vi "Editor UI.vi"(8 "error in (no error)":errorcluster, 11 "Entity Editor in":refnum<class "Entity Editor.lvclass">) -> (0 "error out":errorcluster, 3 "Entity Editor out":refnum<class "Entity Editor.lvclass">)   [LabVIEW 2020, in "Conditum-Tools.lvlib" / "Entity Editor.lvclass"]
uses:
  Entity Editor.lvclass
  Conditum-Clone/Columns/Type/Type.lvclass
  ColumnPanel/ColumnPanel.lvclass
  C:/Program Files (x86)/National Instruments/LabVIEW 2020/vi.lib/IlluminatedG/IG OOPanel/OOPanel/ArrayPanel/ArrayPanel.lvclass
  Conditum-Clone/Columns/Type/Type.lvclass/Type.ctl
  <vilib>/IlluminatedG/IG OOPanel/OOPanel/ArrayManager/ArrayManager.lvclass
  1c4234d0-757c-494a-9175-61bb4fd4687c.vi
  2443108f-0f49-4029-b3c0-d61e9c764f54.vi
  <vilib>/Utility/cursorutil.llb/Set Cursor (Icon Pict).vi
  <vilib>/Utility/LVClass/Get LV Class Name.vi
  <vilib>/Comparison/Equal/Equal Functor/Equal Functor.lvclass
panel:
  out "Project Ref":refnum<vi>
  out "Entity Path":path
  in  "Reset Entity":bool
  in  "Save Entity":bool
  in  "Fields":i32(listbox)
  out "Definition":refnum<class "Type.lvclass">[](array[class])
  out "Target Entity Paths":path[](array[path])
  in  "Refresh Targets":bool
  in  "Target":string(combo)
  in  "Refresh Projects":bool
  in  "New Entity":bool
  in  "Remove Field":bool
  in  "Add Field":bool
  in  "Entity":i32(listbox)
  in  "Project":string(combo)
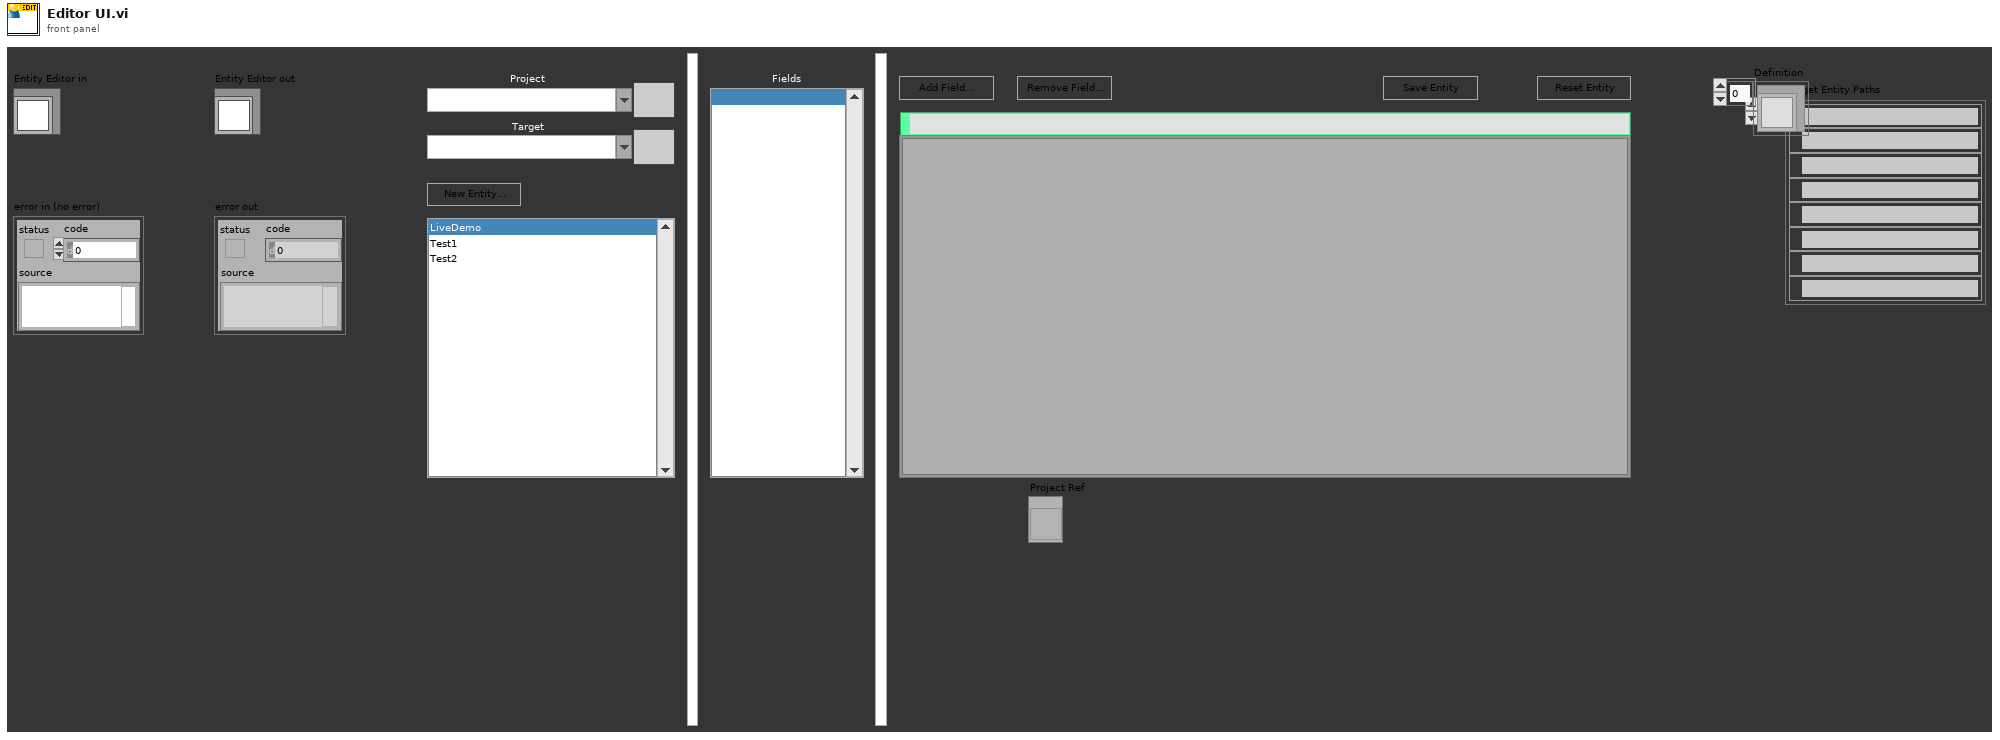
[diagram p1: front panel]
types:
  T1 = typedef "Conditu2.lvlib/Field Type.ctl" = enum16{"None", "ID", "Boolean", "Integer", "Double", "Timestamp", "String", "Text", "Entity"}
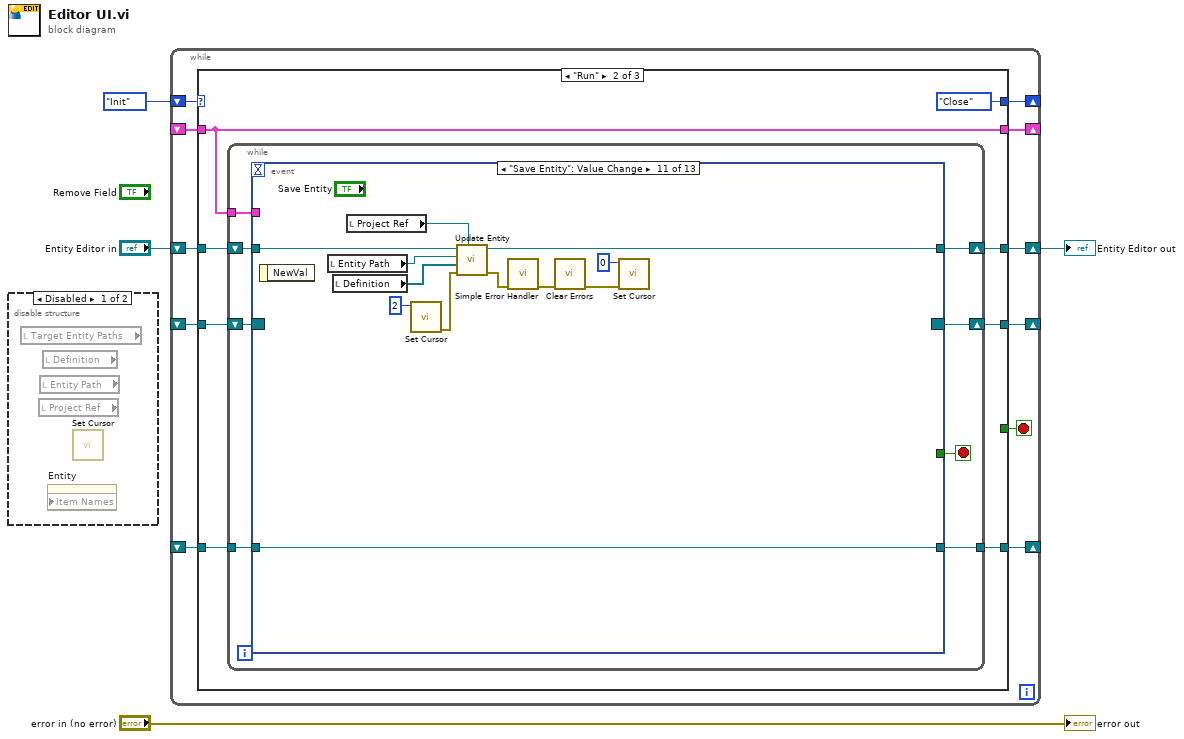
[diagram p0: block diagram]
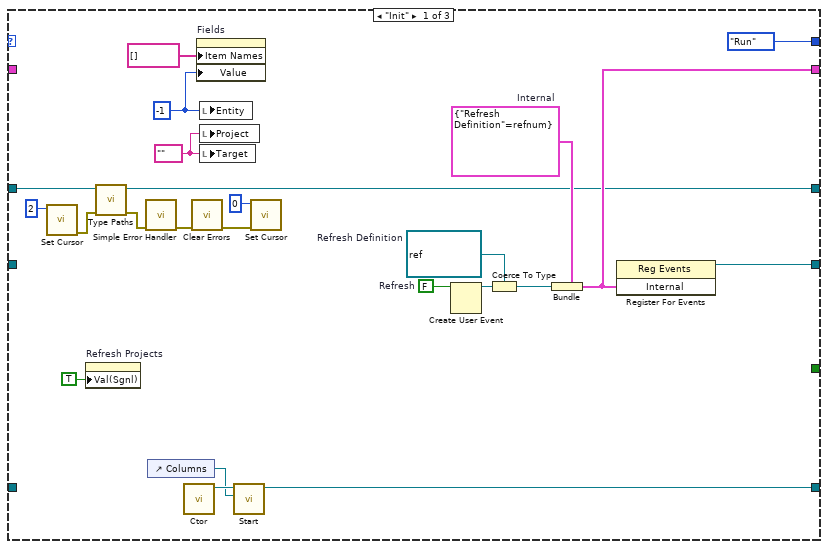
[diagram p3: hidden frame]
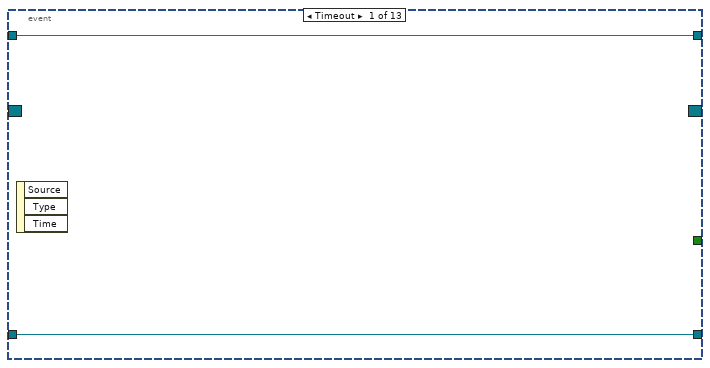
[diagram p4: hidden frame]
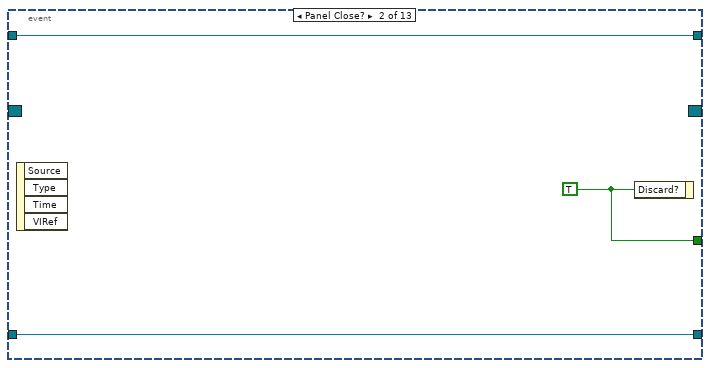
[diagram p5: hidden frame]
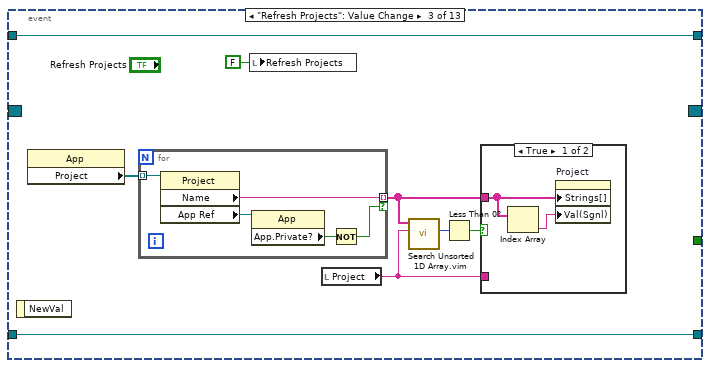
[diagram p6: hidden frame]
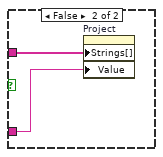
[diagram p7: hidden frame]
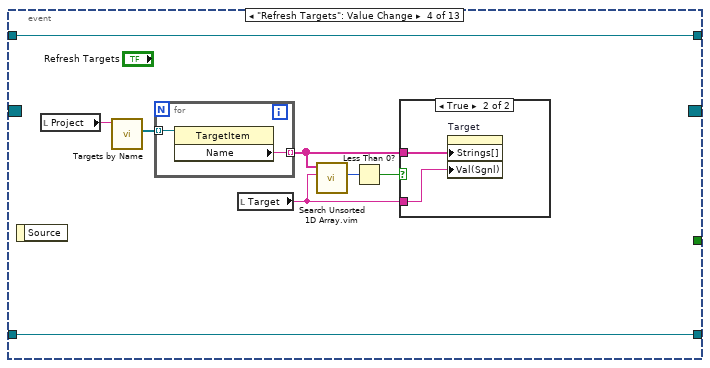
[diagram p8: hidden frame]
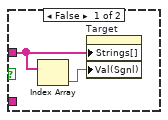
[diagram p9: hidden frame]
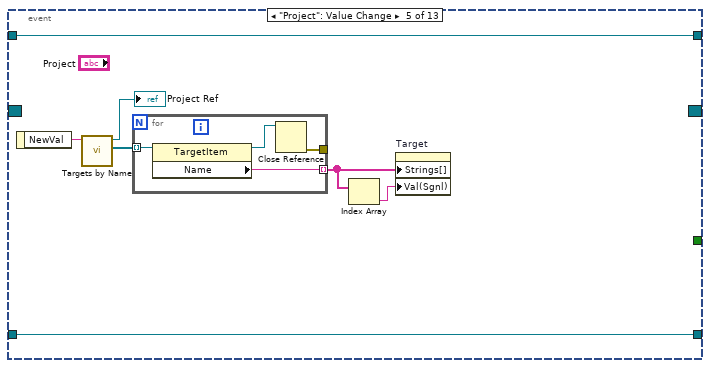
[diagram p10: hidden frame]
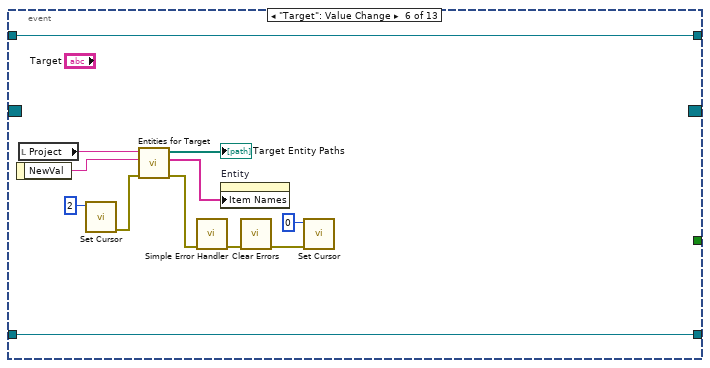
[diagram p11: hidden frame]
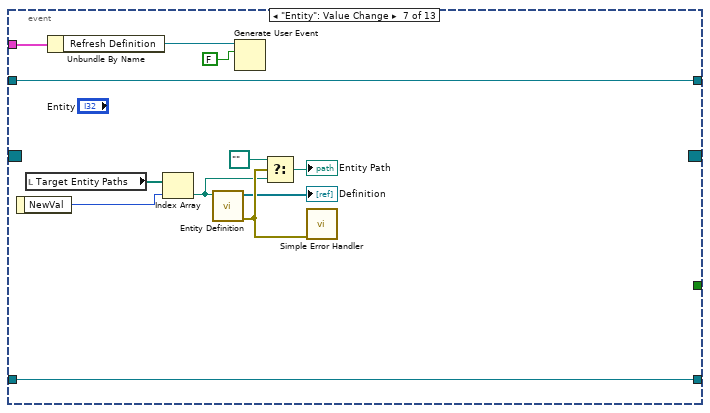
[diagram p12: hidden frame]
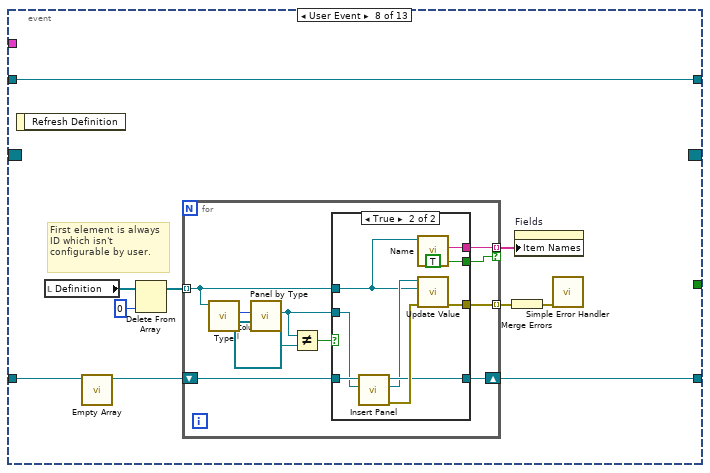
[diagram p13: hidden frame]
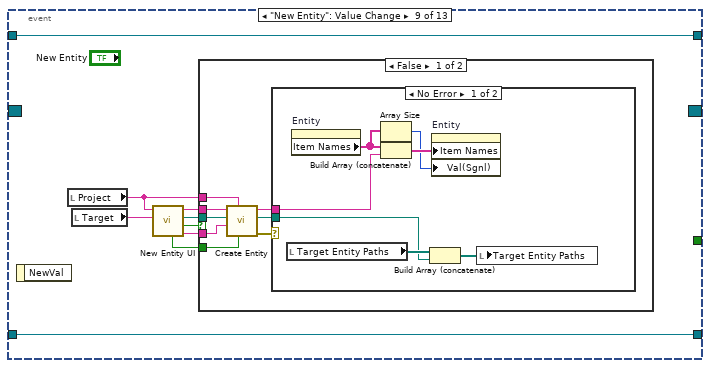
[diagram p15: hidden frame]
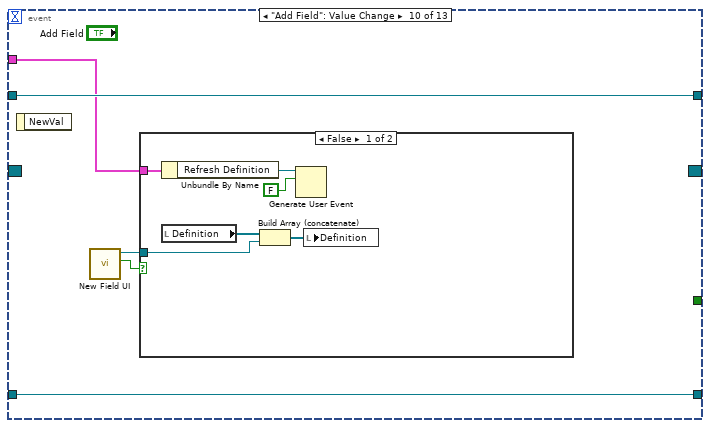
[diagram p18: hidden frame]
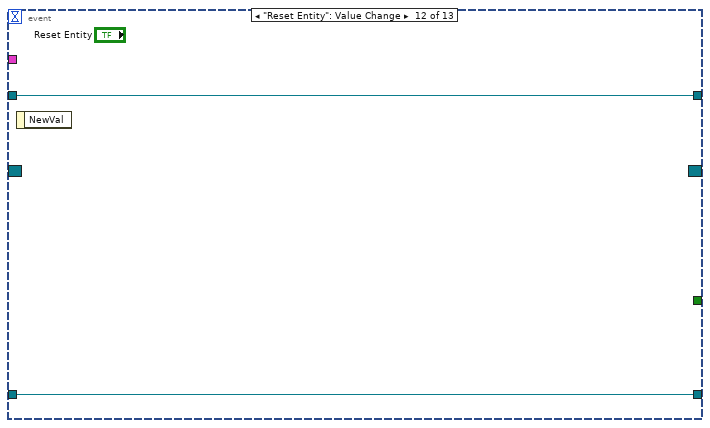
[diagram p20: hidden frame]
diagram:
  n1 = disable-structure shown="Disabled" {
    frame Disabled {
      n2 = local read "Target Entity Paths"() -> ()  [unwired: 1 out]
      n3 = local read "Project Ref"() -> ()  [unwired: 1 out]
      n4 = local read "Entity Path"() -> ()  [unwired: 1 out]
      n5 = local read "Definition"() -> ()  [unwired: 1 out]
      n6 = property on="Entity" class="LstBox (strict)" props=["Item Names"]() -> ()  [unwired: 3 in, 2 out]
      n7 = call-poly <vilib>:"Set Cursor.vi"() -> ()  [unwired: 10 in, 2 out]
    }
    frame Enabled {
    }
  }
  n8 = while {
    shift-right: [w14] -> _
    shift-left: enum16{"Init", "Run", "Close"}."Init" ("Basic UI State") -> [w15]
    shift-right: [w12] -> w2
    shift-left: "Entity Editor in" -> [w13]
    shift-right: [w10] -> _
    shift-left: _ -> [w9]
    shift-right: [w8] -> _
    shift-left: _ -> [w7]
    shift-right: [w6] -> _
    shift-left: _ -> [w5]
    stop <- w11 stop-if-true
    n9 = case shown="\"Run\"" w15 {
      selector: w15 -> [_ _ w216]
      tunnel: [enum16{"Init", "Run", "Close"}."Run" ("Basic UI State") enum16{"Init", "Run", "Close"}."Close" ("Basic UI State") w216] -> w14
      tunnel: w13 -> [w24 w45 w215]
      tunnel: [w23 w44 w215] -> w12
      tunnel: [_ _ TRUE] -> w11
      tunnel: [w31 w42 refnum<class "ArrayManager.lvclass"> refnum ("ArrayManager out")] -> w10
      tunnel: w9 -> [_ w43 w213]
      tunnel: [w27 w40 _] -> w8
      tunnel: w7 -> [_ w41 w209]
      tunnel: [w28 w39 _] -> w6
      tunnel: w5 -> [_ w39 w211]
      frame "Init" {
        w21 = "" ("Target")
        w25 = -1 ("Entities")
        w29 = cluster{"Refresh Definition":refnum<user-event>} {"Refresh Definition"=refnum}  # Internal
        w33 = refnum<user-event> refnum  # Refresh Definition
        w35 = FALSE  # Refresh
        n10 = call-poly <vilib>:"Set Cursor.vi"("icon"=u16 2) -> ("error out"=w19:errorcluster)  [unwired: 9 in, 1 out]
        n11 = property on="Refresh Projects" class="Bool (strict)"("Val(Sgnl)"=TRUE ("Value (Signaling)")) -> ()  [unwired: 2 in, 2 out]
        n12 = call "Type Paths.vi"("error in (no error)"=w19, "Editor in"=w24) -> ("error out"=w22:errorcluster, "Editor out"=w23:refnum<class "Entity Editor.lvclass">)  [unwired: 8 in]
        n13 = call <vilib>:"Simple Error Handler.vi"("error in (no error)"=w22) -> ("error out"=w18:errorcluster)  [unwired: 4 in, 4 out]
        n14 = control-ref of="Columns"() -> (w36:refnum<vi>)
        n15 = call <vilib>:"Ctor.vi"() -> ("PanelArray"=w37:refnum<class "ArrayManager.lvclass">)  [unwired: 10 in, 1 out]
        n16 = call <vilib>:"Clear Errors.vi"("error in (no error)"=w18) -> ("error out"=w17:errorcluster)  [unwired: 5 in, 1 out]
        n17 = property on="Fields" class="LstBox (strict)"("Item Names"=string[] [], "Value"=w25) -> ()  [unwired: 2 in, 2 out]
        n18 = local write "Entity"(w25) -> ()
        n19 = local write "Project"(w21) -> ()
        n20 = local write "Target"(w21) -> ()
        n21 = call <vilib>:"Start.vi"("Container"=w36, "ArrayManager in"=w37) -> ("ArrayManager out"=w31:refnum<class "ArrayManager.lvclass">)  [unwired: 8 in, 1 out]
        n22 = call-poly <vilib>:"Set Cursor.vi"("error in (no error)"=w17, "icon"=u16 0) -> ()  [unwired: 8 in, 2 out]
        n23 = Create User Event(user event datatype=w35) -> (user event=w34:refnum<user-event>)  [unwired: 1 in, 1 out]
        n24 = Coerce To Type(0:w34, 1:w33) -> (2:w32:refnum<user-event>)
        n25 = Bundle(cluster=w29, "Refresh Definition"=w32) -> (w28:cluster{"Refresh Definition":refnum<user-event>})
        n26 = register-events(w28) -> (reference out=w27:refnum<event-registration>)  [unwired: 2 in, 1 out]
      }
      frame "Run" {
        n27 = while {
          shift-right: [w54] -> w44
          shift-left: w45 -> [w53]
          tunnel: w43 -> [w51]
          tunnel: [w50] -> w42
          shift-right: [w49] -> w40
          shift-left: w41 -> [w47]
          tunnel: w39 -> [w48]
          stop <- w52 stop-if-true
          n28 = event shown="[10] \"Save Entity\": Value Change" {
            selector: w47 -> [_ _ _ _ _ _ _ _ _ _ _ _ _]
            dyn-events: [_ _ _ _ _ _ _ _ _ _ _ _ _] -> w49
            timeout: _ -> [_ _ _ _ _ _ _ _ _ _ _ _ _]
            tunnel: [w56 w59 w67 w84 w97 w113 w124 w135 w161 w181 w200 w204 w208] -> w54
            tunnel: w53 -> [w56 w59 w67 w84 w97 w113 w124 w135 w161 w181 w201 w204 w208]
            tunnel: [_ w58 _ _ _ _ _ _ _ _ _ _ _] -> w52
            tunnel: w51 -> [w55 w57 w66 w83 w96 w112 w123 w131 w164 w184 w202 w203 w206]
            tunnel: [w55 w57 w66 w83 w96 w112 w123 w129 w164 w184 w202 w203 w206] -> w50
            tunnel: w48 -> [_ _ _ _ _ _ w120 _ _ w180 _ _ _]
            event Timeout {
              n29 = event-data() -> ()  [unwired: 1 in, 3 out]
            }
            event Panel Close? {
              w58 = TRUE ("Discard?")
              n30 = event-data() -> ()  [unwired: 1 in, 4 out]
              n31 = event-data("Discard?"=w58) -> ()  [unwired: 1 in, 1 out]
            }
            event "Refresh Projects": Value Change {
              n32 = event-data() -> ()  [unwired: 1 in, 1 out]
              n33 = property class="App"() -> ("Project"=w64:refnum<vi>[])  [unwired: 2 in, 2 out]
              n34 = for {
                tunnel: w64 -> [w76] mode=indexing
                tunnel: [w73] -> w63 mode=indexing if=w72
                n35 = property class="Project"(reference=w76) -> ("Name"=w73:string, "App Ref"=w75:refnum<vi>)  [unwired: 1 in, 2 out]
                n36 = property class="App"(reference=w75) -> ("App.Private?"=w74:bool)  [unwired: 1 in, 2 out]
                n37 = Not(x=w74) -> (.not. x?=w72:bool)
              }
              n38 = local write "Refresh Projects"(FALSE ("Refresh Projects")) -> ()
              n39 = local read "Project"() -> (w60:string)
              n40 = call "Search Unsorted 1D Array.vim"("element"=w60, "unsorted 1D array"=w63) -> ("index of element"=w62:i32)  [unwired: 9 in]
              n41 = Less Than 0?(x=w62) -> (x < 0?=w61:bool)
              n42 = case shown="True" w61 {
                tunnel: w63 -> [w69 w71]
                tunnel: w60 -> [_ w70]
                frame True {
                  n43 = Index Array(array=w69) -> (element=w68:string)  [unwired: 1 in]
                  n44 = property on="Project" class="CmbBox"("Strings[]"=w69, "Val(Sgnl)"=w68) -> ()  [unwired: 2 in, 2 out]
                }
                frame False {
                  n45 = property on="Project" class="CmbBox"("Strings[]"=w71, "Value"=w70) -> ()  [unwired: 2 in, 2 out]
                }
              }
            }
            event "Refresh Targets": Value Change {
              n46 = event-data() -> ()  [unwired: 1 in, 1 out]
              n47 = local read "Project"() -> (w81:string)
              n48 = call "Targets by Name.vi"("Project Name"=w81) -> ("Targets"=w82:refnum<vi>[])  [unwired: 9 in, 1 out]
              n49 = for {
                tunnel: w82 -> [w90] mode=indexing
                tunnel: [w89] -> w78 mode=indexing
                n50 = property class="TargetItem"(reference=w90) -> ("Name"=w89:string)  [unwired: 1 in, 2 out]
              }
              n51 = local read "Target"() -> (w77:string)
              n52 = call "Search Unsorted 1D Array.vim"("element"=w77, "unsorted 1D array"=w78) -> ("index of element"=w80:i32)  [unwired: 9 in]
              n53 = Less Than 0?(x=w80) -> (x < 0?=w79:bool)
              n54 = case shown="True" w79 {
                tunnel: w78 -> [w86 w88]
                tunnel: w77 -> [_ w87]
                frame False {
                  n55 = Index Array(array=w86) -> (element=w85:string)  [unwired: 1 in]
                  n56 = property on="Target" class="CmbBox"("Strings[]"=w86, "Val(Sgnl)"=w85) -> ()  [unwired: 2 in, 2 out]
                }
                frame True {
                  n57 = property on="Target" class="CmbBox"("Strings[]"=w88, "Val(Sgnl)"=w87) -> ()  [unwired: 2 in, 2 out]
                }
              }
            }
            event "Project": Value Change {
              n58 = event-data() -> ("NewVal"=w95:string)  [unwired: 1 in]
              n59 = call "Targets by Name.vi"("Project Name"=w95) -> ("Targets"=w94:refnum<vi>[], "Project"=→"Project Ref":refnum<vi>)  [unwired: 9 in]
              n60 = for {
                tunnel: w94 -> [w101] mode=indexing
                tunnel: [w100] -> w93 mode=indexing
                tunnel: [w98] -> _
                n61 = property class="TargetItem"(reference=w101) -> (reference out=w99:refnum<vi>, "Name"=w100:string)  [unwired: 1 in, 1 out]
                n62 = Close Reference(reference=w99) -> (error out=w98:errorcluster)  [unwired: 1 in]
              }
              n63 = Index Array(array=w93) -> (element=w92:string)  [unwired: 1 in]
              n64 = property on="Target" class="CmbBox"("Strings[]"=w93, "Val(Sgnl)"=w92) -> ()  [unwired: 2 in, 2 out]
            }
            event "Target": Value Change {
              n65 = event-data() -> ("NewVal"=w110:string)  [unwired: 1 in]
              n66 = local read "Project"() -> (w111:string)
              n67 = call-poly <vilib>:"Set Cursor.vi"("icon"=u16 2) -> ("error out"=w106:errorcluster)  [unwired: 9 in, 1 out]
              n68 = call "Entities for Target.vi"("error in (no error)"=w106, "Target Name"=w110, "Project Name"=w111) -> ("error out"=w107:errorcluster, "Names"=w108:string[], "Entities"=→"Target Entity Paths":path[])  [unwired: 6 in]
              n69 = call <vilib>:"Simple Error Handler.vi"("error in (no error)"=w107) -> ("error out"=w104:errorcluster)  [unwired: 4 in, 4 out]
              n70 = property on="Entity" class="LstBox (strict)"("Item Names"=w108) -> ()  [unwired: 2 in, 2 out]
              n71 = call <vilib>:"Clear Errors.vi"("error in (no error)"=w104) -> ("error out"=w102:errorcluster)  [unwired: 5 in, 1 out]
              n72 = call-poly <vilib>:"Set Cursor.vi"("error in (no error)"=w102, "icon"=u16 0) -> ()  [unwired: 8 in, 2 out]
            }
            event "Entity": Value Change {
              n73 = event-data() -> ("NewVal"=w121:i32)  [unwired: 1 in]
              n74 = local read "Target Entity Paths"() -> (w122:path[])
              n75 = Unbundle By Name(w120) -> ("Refresh Definition"=w119:refnum<user-event>)
              n76 = Index Array(array=w122, index=w121) -> (element=w116:path)
              n77 = call "Entity Definition.vi"("Path"=w116) -> ("error out"=w125:errorcluster, "Definition"=→"Definition":refnum<class "Type.lvclass">[])  [unwired: 8 in, 1 out]
              n78 = Generate User Event(user event=w119, event data cluster=FALSE ("event data")) -> ()  [unwired: 2 in, 2 out]
              n79 = Select(t=path "", s=w125, f=w116) -> (s? t:f=→"Entity Path":path)
              n80 = call <vilib>:"Simple Error Handler.vi"("error in (no error)"=w125) -> ()  [unwired: 4 in, 5 out]
            }
            event User Event {
              # "First element is always ID which isn't configurable by user."
              n81 = event-data() -> ()  [unwired: 1 in, 1 out]
              n82 = local read "Definition"() -> (w134:refnum<class "Type.lvclass">[])
              n83 = call <vilib>:"Empty Array.vi"("ArrayManager in"=w131) -> ("ArrayManager out"=w130:refnum<class "ArrayManager.lvclass">)  [unwired: 9 in, 1 out]
              n84 = Delete From Array(array=w134, index=0) -> (array with subset deleted=w133:refnum<class "Type.lvclass">[])  [unwired: 1 in, 1 out]
              n85 = for {
                tunnel: w133 -> [w140] mode=indexing
                shift-right: [w139] -> w129
                shift-left: w130 -> [w143]
                tunnel: [w138] -> w128 mode=indexing
                tunnel: [w137] -> w126 mode=indexing if=w136
                n86 = call "Type.vi"("Type in"=w140) -> ("Type"=w145:T1)  [unwired: 10 in]
                n87 = call "Panel by Type.vi"("Type"=w145) -> ("ColumnPanel"=w141:refnum<class "ColumnPanel.lvclass">)  [unwired: 10 in]
                n88 = Not Equal?(x=w141, y=refnum<class "ColumnPanel.lvclass"> refnum) -> (x != y?=w142:bool)
                n89 = case shown="True" w142 {
                  tunnel: w143 -> [w146 w154]
                  tunnel: w141 -> [_ w153]
                  tunnel: w140 -> [_ w149]
                  tunnel: [w146 w152] -> w139
                  tunnel: [_ w151] -> w138
                  tunnel: [_ w148] -> w137
                  tunnel: [_ TRUE] -> w136
                  frame False {
                  }
                  frame True {
                    n90 = call <vilib>:"Insert Panel.vi"("Panel/Type"=w153, "PanelArray in"=w154) -> ("error out"=w155:errorcluster, "Panel"=w150:refnum<class "ColumnPanel.lvclass">, "PanelArray out"=w152:refnum<class "ArrayManager.lvclass">)  [unwired: 7 in]
                    n91 = call "Name.vi"("Type in"=w149) -> ("Table Name"=w148:string)  [unwired: 10 in]
                    n92 = call "Update Value.vi"("error in (no error)"=w155, "Type Value"=w149, "ColumnPanel in"=w150) -> ("error out"=w151:errorcluster)  [unwired: 7 in, 1 out]
                  }
                }
              }
              n93 = Merge Errors(w128) -> (w127:errorcluster)
              n94 = property on="Fields" class="LstBox (strict)"("Item Names"=w126) -> ()  [unwired: 2 in, 2 out]
              n95 = call <vilib>:"Simple Error Handler.vi"("error in (no error)"=w127) -> ()  [unwired: 4 in, 5 out]
            }
            event "New Entity": Value Change {
              n96 = event-data() -> ()  [unwired: 1 in, 1 out]
              n97 = local read "Project"() -> (w156:string)
              n98 = local read "Target"() -> (w162:string)
              n99 = call "New Entity UI.vi"("Target Name"=w162, "Project Name"=w156) -> ("Container"=w158:string, "Cancelled"=w160:bool, "Folder"=w159:path, "Entity Name"=w163:string, "Library?"=w157:bool)  [unwired: 5 in]
              n100 = case shown="False" w160 {
                tunnel: w163 -> [w167 _]
                tunnel: w159 -> [w172 _]
                tunnel: w158 -> [w171 _]
                tunnel: w157 -> [w169 _]
                tunnel: w156 -> [w170 _]
                frame False {
                  n101 = call "Create Entity.vi"("Library"=w169, "Project"=w170, "Container"=w171, "Folder"=w172, "Entity Name in"=w167) -> ("error out"=w168:errorcluster, "New Entity Path"=w165:path, "Entity Name"=w166:string)  [unwired: 4 in]
                  n102 = case shown="No Error" w168 {
                    tunnel: w166 -> [w179 _]
                    tunnel: w165 -> [w176 _]
                    frame No Error {
                      n103 = local read "Target Entity Paths"() -> (w177:path[])
                      n104 = property on="Entity" class="LstBox (strict)"() -> ("Item Names"=w174:string[])  [unwired: 2 in, 2 out]
                      n105 = Array Size(array=w174) -> (size(s)=w173:i32)
                      n106 = Build Array (concatenate)(w174, w179) -> (w178:string[])
                      n107 = Build Array (concatenate)(w177, w176) -> (w175:path[])
                      n108 = property on="Entity" class="LstBox (strict)"("Item Names"=w178, "Val(Sgnl)"=w173) -> ()  [unwired: 2 in, 2 out]
                      n109 = local write "Target Entity Paths"(w175) -> ()
                    }
                    frame Error {
                    }
                  }
                }
                frame True {
                }
              }
            }
            event "Add Field": Value Change {
              n110 = event-data() -> ()  [unwired: 1 in, 1 out]
              n111 = call "New Field UI.vi"() -> ("Cancelled"=w183:bool, "Field"=w182:refnum<class "Type.lvclass">)  [unwired: 10 in]
              n112 = case shown="False" w183 {
                tunnel: w182 -> [w189 _]
                tunnel: w180 -> [w187 _]
                frame False {
                  n113 = Unbundle By Name(w187) -> ("Refresh Definition"=w186:refnum<user-event>)
                  n114 = local read "Definition"() -> (w190:refnum<class "Type.lvclass">[])
                  n115 = Build Array (concatenate)(w190, w189) -> (w188:refnum<class "Type.lvclass">[])
                  n116 = Generate User Event(user event=w186, event data cluster=FALSE ("event data")) -> ()  [unwired: 2 in, 2 out]
                  n117 = local write "Definition"(w188) -> ()
                }
                frame True {
                }
              }
            }
            event "Save Entity": Value Change {
              n118 = event-data() -> ()  [unwired: 1 in, 1 out]
              n119 = local read "Entity Path"() -> (w199:path)
              n120 = local read "Definition"() -> (w198:refnum<class "Type.lvclass">[])
              n121 = local read "Project Ref"() -> (w196:refnum<vi>)
              n122 = call-poly <vilib>:"Set Cursor.vi"("icon"=u16 2) -> ("error out"=w191:errorcluster)  [unwired: 9 in, 1 out]
              n123 = call "Update Entity.vi"("Project Ref"=w196, "error in (no error)"=w191, "Definition"=w198, "Entity Path"=w199, "Entity Editor in"=w201) -> ("error out"=w197:errorcluster, "Entity Editor out"=w200:refnum<class "Entity Editor.lvclass">)  [unwired: 5 in]
              n124 = call <vilib>:"Simple Error Handler.vi"("error in (no error)"=w197) -> ("error out"=w195:errorcluster)  [unwired: 4 in, 4 out]
              n125 = call <vilib>:"Clear Errors.vi"("error in (no error)"=w195) -> ("error out"=w194:errorcluster)  [unwired: 5 in, 1 out]
              n126 = call-poly <vilib>:"Set Cursor.vi"("error in (no error)"=w194, "icon"=u16 0) -> ()  [unwired: 8 in, 2 out]
            }
            event "Reset Entity": Value Change {
              n127 = event-data() -> ()  [unwired: 1 in, 1 out]
            }
            event "Fields": Value Change {
              n128 = event-data() -> ("NewVal"=w207:i32)  [unwired: 1 in]
              n129 = call <vilib>:"Scroll Panel Into View.vi"("Highlight (F)"=TRUE, "Panel Index"=w207, "ArrayManager in"=w206) -> ()  [unwired: 7 in, 2 out]
            }
          }
        }
      }
      frame "Close" {
        n130 = Unregister For Events(event registration refnum=w209) -> ()  [unwired: 1 in, 1 out]
        n131 = call <vilib>:"Cleanup.vi"("PanelArray in"=w213) -> ()  [unwired: 10 in, 1 out]
        n132 = Unbundle By Name(w211) -> ("Refresh Definition"=w210:refnum<user-event>)
        n133 = Destroy User Event(user event=w210) -> ()  [unwired: 1 in, 1 out]
      }
    }
  }
  "Entity Editor out" <- w2
  "error out" <- "error in (no error)"
